vi "Set Start Trigger Options.vi"(8 "error in (no error)":errorcluster, 9 "Retriggerable":bool, 10 "Pre-Trigger Duration":dbl, 11 "Data Logging Specification Ref in":T1) -> (0 "error out":errorcluster, 3 "Data Logging Specification Ref out":T1)   [LabVIEW 2020, in "NI_VS Data Logging API.lvlib"]
doc: "Sets common start trigger options."
uses:
  <vilib>/NI VeriStand/Execution/DataLogging/NI_VS Data Logging API.lvlib
  <vilib>/NI VeriStand/Execution/DataLogging/DataLoggingSpecification Ref.ctl
  NationalInstruments.VeriStand.ClientAPI
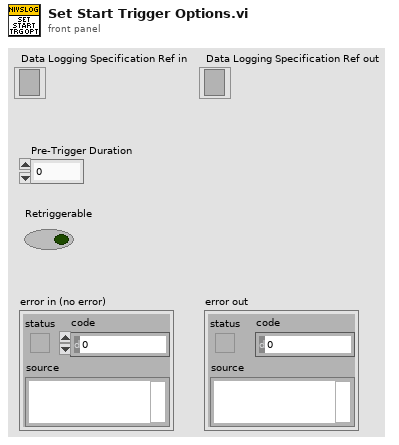
[diagram p1: front panel]
types:
  T1 = typedef "NI_VS Data Logging API.lvlib/DataLoggingSpecification Ref.ctl" = refnum<k24>
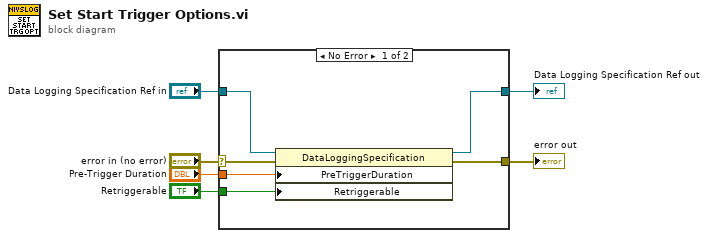
[diagram p0: block diagram]
diagram:
  n1 = case shown="No Error" "error in (no error)" {
    selector: "error in (no error)" -> [w9 w13]
    tunnel: [w12 w13] -> w6
    tunnel: [w11 w14] -> w5
    tunnel: "Data Logging Specification Ref in" -> [w10 w14]
    tunnel: "Pre-Trigger Duration" -> [w8 _]
    tunnel: "Retriggerable" -> [w7 _]
    frame No Error {
      n2 = property class="DataLoggingSpecification"(reference=w10, error in=w9, "PreTriggerDuration"=w8, "Retriggerable"=w7) -> (reference out=w11:T1, error out=w12:errorcluster)
    }
    frame Error {
    }
  }
  "error out" <- w6
  "Data Logging Specification Ref out" <- w5
